vi "确定当前的指令名称.vi"(1 "索引":i32) -> (0 "指令名称":string)   [LabVIEW 2015]
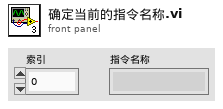
[diagram p1: front panel]
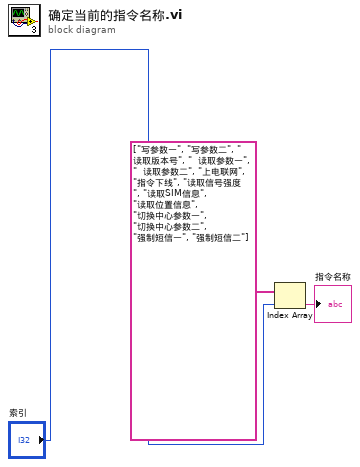
[diagram p0: block diagram]
diagram:
  n1 = Index Array(array=string[] ["写参数一", "写参数二", "  读取版本号", "  读取参数一", "  读取参数二", "上电联网", "指令下线", "读取信号强度   ", "读取SIM信息", "读取位置信息", "切换中心参数一", "切换中心参数二", "强制短信一", "强制短信二"], index="索引") -> (element=→"指令名称":string)
